vi "IMAQdx HL-Snap.vi"(8 "ErrIn":errorcluster) -> (0 "ErrOut":errorcluster)   [LabVIEW 2020]
doc: "Use this template to build a VI to use as a subVI."
uses:
  <vilib>/userDefined/High Color/IMAQdx.ctl
  <vilib>/vision/driver/NI_Vision_Acquisition_Software.lvlib
panel:
  in  "Camera":T1="cam1"
  out "Image":T2(plugin-control)
  # "Output Image"
  # "Input Parameters"
  # "Instruction:\n1) Select the camera device;\n2) Rund VI and see the snapped image."
  # "VI Description:\nThis VI is created to snap a image from imaging device."
  # ":: MVI Framework V1.0 ::\nAuthor:Gaoke Yang\nEmail: gaoke.yang@yahoo.com\nWeb: www.mvicontrol.com\nCopyright (C) 2013, MVI Technologies All Rights Reserved"
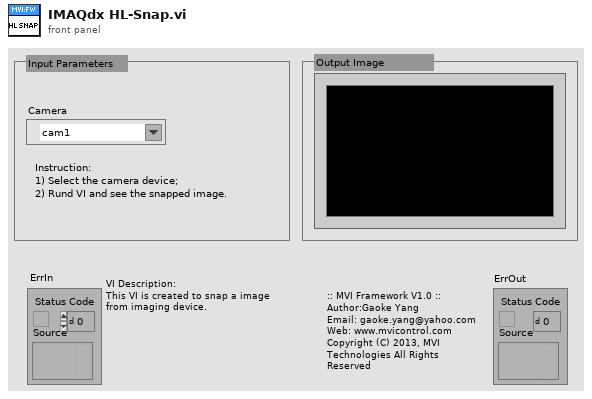
[diagram p1: front panel]
types:
  T1 = typedef "IMAQdx.ctl" = refnum<k21>
  T2 = typedef "IMAQ Image.ctl" = refnum<image>
  T3 = typedef "Image Type" = u32
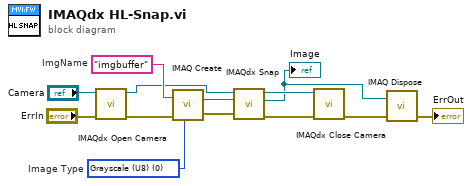
[diagram p0: block diagram]
diagram:
  w1 = T3 0 items=["Grayscale (U8)", "Grayscale (I16)", "Grayscale (SGL)", "Complex (CSG)", "RGB (U32)", "HSL (U32)", "RGB (U64)", "Grayscale (U16)"]  # Image Type
  w12 = "imgbuffer"  # ImgName
  n1 = call <vilib>:"IMAQdx Open Camera.vi"("error in"="ErrIn", "Session In"="Camera") -> ("error out"=w4:errorcluster, "Session Out"=w3:T1)  [unwired: 8 in]
  n2 = call "IMAQ Create"("Image Name"=w12, "Image Type"=w1, "error in (no error)"=w4) -> ("New Image"=w9:T2, "error out"=w8:errorcluster)  [unwired: 1 in, 1 out]
  n3 = call <vilib>:"IMAQdx Snap.vi"("error in"=w8, "Image In"=w9, "Session In"=w3) -> ("error out"=w5:errorcluster, "Image Out"=w2:T2, "Session Out"=w6:T1)  [unwired: 6 in]
  "Image" <- w2
  n4 = call <vilib>:"IMAQdx Close Camera.vi"("error in"=w5, "Session In"=w6) -> ("error out"=w7:errorcluster)  [unwired: 9 in]
  n5 = call "IMAQ Dispose"("Image"=w2, "error in (no error)"=w7) -> ("error out"=→"ErrOut":errorcluster)  [unwired: 1 in, 3 out]
